vi "ReadPos.vi"(8 "error in (no error)":errorcluster, 11 "XuLyStringUART in":refnum<class "XuLyStringUART.lvclass">) -> (0 "error out":errorcluster, 3 "XuLyStringUART out":refnum<class "XuLyStringUART.lvclass">)   [LabVIEW 2017, in "LibraryGcode.lvlib" / "XuLyStringUART.lvclass"]
uses:
  XuLyStringUART.lvclass
  control/stateBoardFirmware.ctl
  XuLyStringUART.lvclass/XuLyStringUART.ctl
  LibraryGcode.lvlib
panel:
  out "outPOS":T2
  out "output 1":string
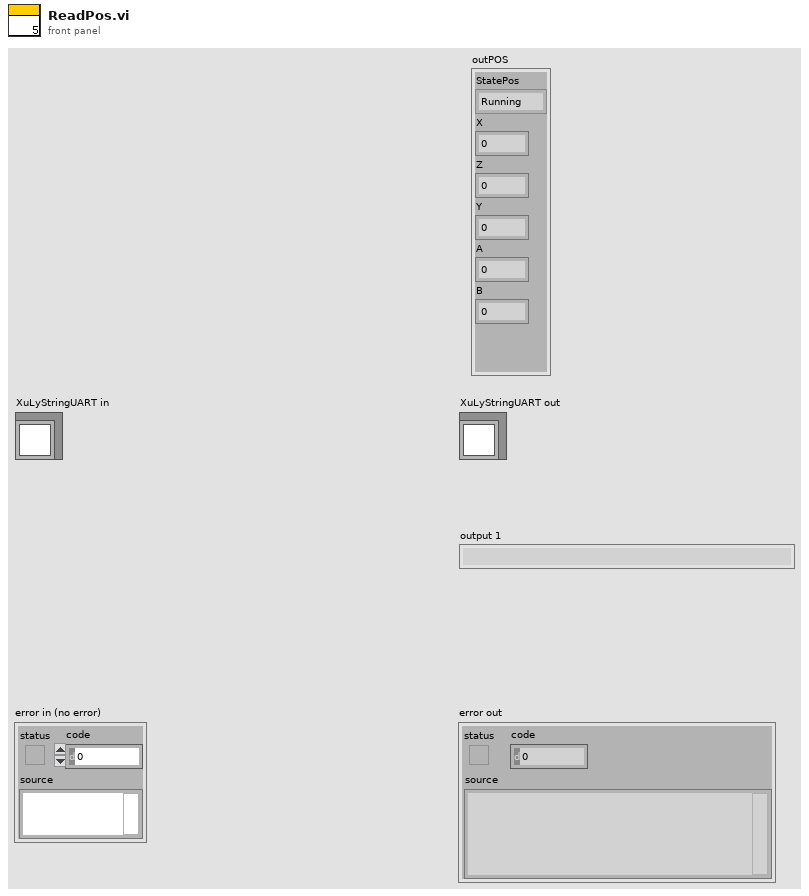
[diagram p1: front panel]
types:
  T1 = typedef "LibraryGcode.lvlib/stateBoardFirmware.ctl" = enum16{"Running", "Waiting", "Pos", "IDLE"}
  T2 = cluster{"StatePos":T1, "X":dbl, "Z":dbl, "Y":dbl, "A":dbl, "B":dbl}
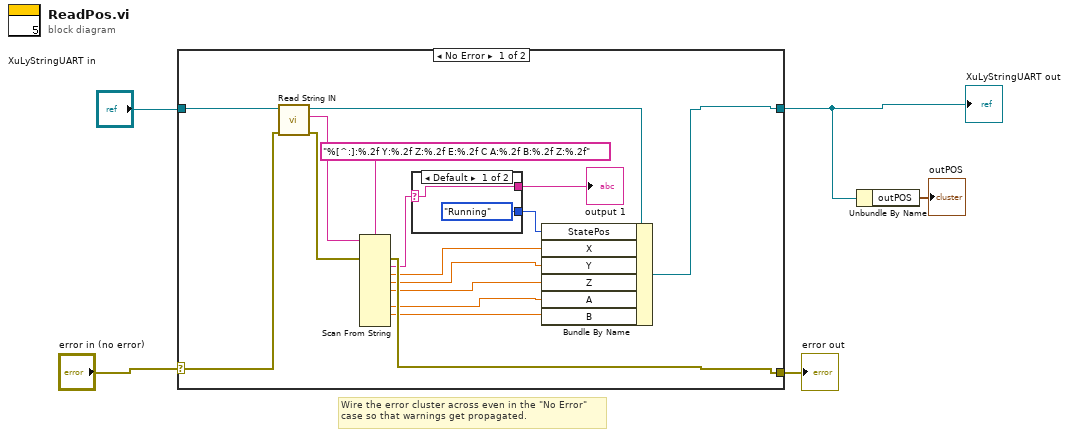
[diagram p0: block diagram]
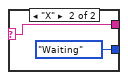
[diagram p2: hidden frame]
diagram:
  # "Wire the error cluster across even in the \"No Error\"\ncase so that warnings get propagated."
  n1 = case shown="No Error" "error in (no error)" {
    selector: "error in (no error)" -> [w19 w27]
    tunnel: [w20 w27] -> w4
    tunnel: [w6 w26] -> w3
    tunnel: "XuLyStringUART in" -> [w21 w26]
    frame No Error {
      n2 = call-dynamic "Read String IN.vi"("error in (no error)"=w19, "XuLyStringUART in"=w21) -> ("error out"=w13:errorcluster, "String IN"=w12:string, "XuLyStringUART out"=w14:refnum<class "XuLyStringUART.lvclass">)  [unwired: 7 in]
      n3 = Scan From String(format string="%[^:]:%.2f Y:%.2f Z:%.2f E:%.2f C A:%.2f B:%.2f Z:%.2f", input string=w12, error in=w13) -> (error out=w20:errorcluster, output 1=w9:string, output 2=w11:dbl, output 3=w10:dbl, output 4=w16:dbl, output 6=w17:dbl, output 7=w18:dbl)  [unwired: 11 in, 2 out]
      n4 = case shown="Default" w9 {
        selector: w9 -> [w22 w24]
        tunnel: [stateBoardFirmware."Running" ("outPOS.StatePos") stateBoardFirmware."Waiting" ("outPOS.StatePos")] -> w8
        tunnel: [w22 w24] -> w7
        frame Default {
        }
        frame "X" {
        }
      }
      "output 1" <- w7
      n5 = Bundle By Name(cluster=w14, "StatePos"=w8, "X"=w11, "Y"=w10, "Z"=w16, "A"=w17, "B"=w18) -> (w6:refnum<class "XuLyStringUART.lvclass">)
    }
    frame Error {
    }
  }
  "error out" <- w4
  "XuLyStringUART out" <- w3
  n6 = Unbundle By Name(w3) -> ("outPOS"=→"outPOS":T2)
